vi "sub_waypoint_resample.vi"(11 "line point":cluster{dbl, dbl}[](array[cluster])) -> (2 "distance":dbl format="%.2f", 3 "interpolate 1d array":cluster{dbl, dbl}[](array[cluster]))   [LabVIEW 2019]
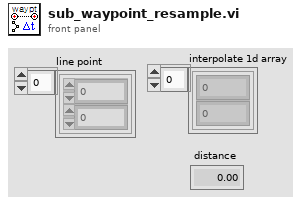
[diagram p1: front panel]
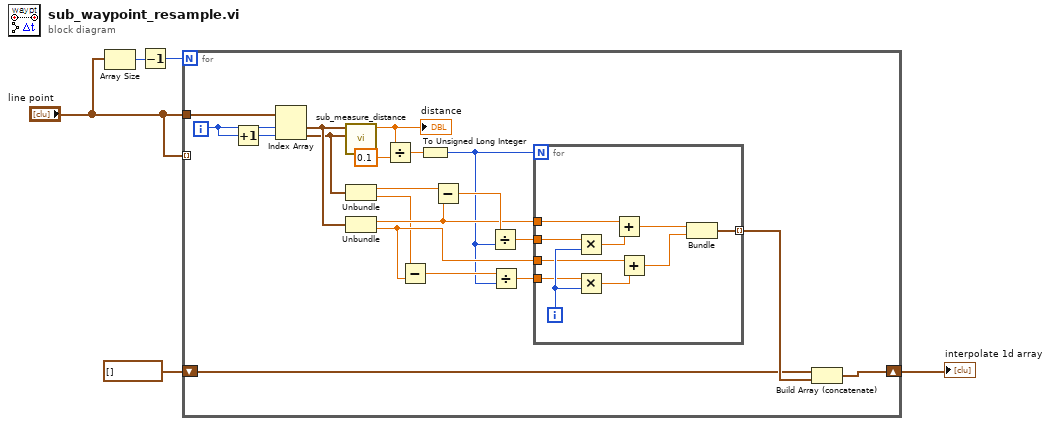
[diagram p0: block diagram]
diagram:
  n1 = Array Size(array="line point") -> (size(s)=w2:i32)
  n2 = Decrement(x=w2) -> (x-1=w1:i32)
  n3 = for {
    N: w1 -> [_]
    tunnel: "line point" -> [w11]
    tunnel: "line point" -> [_] mode=indexing
    shift-right: [w6] -> w4
    shift-left: cluster{dbl, dbl}[] [] -> [w7]
    i -> [w10]
    n4 = Increment(x=w10) -> (x+1=w9:i32)
    n5 = Index Array(array=w11, index #1=w10, index #2=w9) -> (element #1=w21:cluster{dbl, dbl}, element #2=w20:cluster{dbl, dbl})
    n6 = call "sub_measure_distance.vi"("pt 2"=w20, "pt 1"=w21) -> ("distance"=w12:dbl)  [unwired: 9 in]
    "distance" <- w12
    n7 = Unbundle(w20) -> (w15:dbl, w19:dbl)
    n8 = Unbundle(w21) -> (w22:dbl, w25:dbl)
    n9 = Divide(x=w12, y=0.1) -> (x/y=w14:dbl)
    n10 = Subtract(x=w19, y=w25) -> (x-y=w18:dbl)
    n11 = To Unsigned Long Integer(number=w14) -> (unsigned 32bit integer=w17:u32)
    n12 = Subtract(x=w15, y=w22) -> (x-y=w24:dbl)
    n13 = Divide(x=w24, y=w17) -> (x/y=w16:dbl)
    n14 = Divide(x=w18, y=w17) -> (x/y=w23:dbl)
    n15 = for {
      N: w17 -> [_]
      tunnel: w22 -> [w35]
      tunnel: w16 -> [w33]
      tunnel: w25 -> [w30]
      tunnel: w23 -> [w29]
      tunnel: [w26] -> w8 mode=indexing
      i -> [w31]
      n16 = Multiply(x=w33, y=w31) -> (x*y=w34:dbl)
      n17 = Multiply(x=w29, y=w31) -> (x*y=w32:dbl)
      n18 = Add(x=w35, y=w34) -> (x+y=w27:dbl)
      n19 = Add(x=w30, y=w32) -> (x+y=w28:dbl)
      n20 = Bundle(w27, w28) -> (w26:cluster{dbl, dbl})  [unwired: 1 in]
    }
    n21 = Build Array (concatenate)(w7, w8) -> (w6:cluster{dbl, dbl}[])
  }
  "interpolate 1d array" <- w4
